vi "testScopeBasic.vi"() -> ()   [LabVIEW 2023, in "sweScope.lvlib"]
doc: "Demonstrates the usage of the Scope abstraction."
uses:
  sweScope.lvlib
  Data/scopeChnCoupling.ctl
  Data/scopeEdgeTrigger.ctl
  Data/scopeRunState.ctl
  Scope.lvclass
panel:
  out "Waveform Graph":waveform(dbl)(graph)
  out "error out":errorcluster
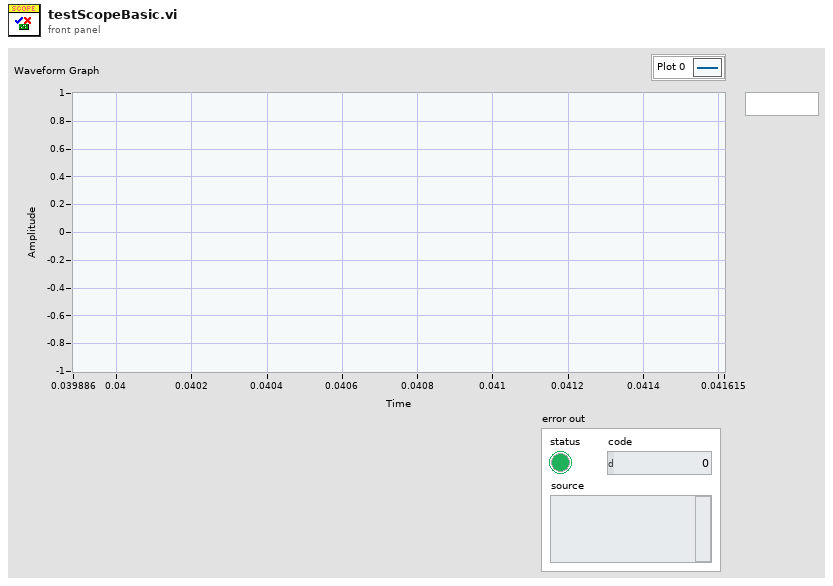
[diagram p1: front panel]
types:
  T1 = typedef "sweScope.lvlib/scopeRunState.ctl" = enum16{"AUTO", "NORMAL", "SINGLE"}
  T2 = typedef "sweScope.lvlib/scopeEdgeTrigger.ctl" = enum16{"Positive", "Negative", "Either"}
  T3 = typedef "sweScope.lvlib/scopeChnCoupling.ctl" = enum16{"DC1M", "AC1M", "DC50", "GND"}
  T4 = enum16{"Simulated", "SCOPE_NI", "SCOPE_Keysight"}
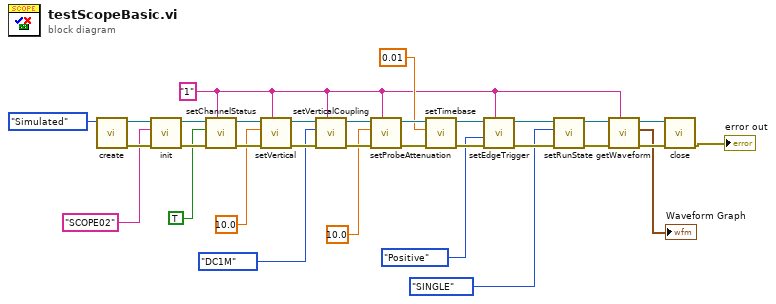
[diagram p0: block diagram]
diagram:
  w6 = "1" ("Chn")
  n1 = call "create.vi"("Type"=T4."Simulated") -> ("error out"=w31:errorcluster, "Scope.lvclass"=w32:refnum<class "Scope.lvclass">)  [unwired: 9 in]
  n2 = call-dynamic "init.vi"("error in (no error)"=w31, "Resource"="SCOPE02", "Instrument in"=w32) -> ("error out"=w29:errorcluster, "Instrument out"=w30:refnum<class "Scope.lvclass">)  [unwired: 7 in]
  n3 = call-dynamic "setChannelStatus.vi"("Chn"=w6, "error in (no error)"=w29, "State"=TRUE, "Scope in"=w30) -> ("error out"=w27:errorcluster, "Scope out"=w28:refnum<class "Scope.lvclass">)  [unwired: 6 in]
  n4 = call-dynamic "setVertical.vi"("Chn"=w6, "error in (no error)"=w27, "Range [V]"=10.0, "Scope in"=w28) -> ("error out"=w25:errorcluster, "Scope out"=w26:refnum<class "Scope.lvclass">)  [unwired: 6 in]
  n5 = call-dynamic "setVerticalCoupling.vi"("Chn"=w6, "error in (no error)"=w25, "Coupling"=scopeChnCoupling."DC1M", "Scope in"=w26) -> ("error out"=w23:errorcluster, "Scope out"=w24:refnum<class "Scope.lvclass">)  [unwired: 6 in]
  n6 = call-dynamic "setProbeAttenuation.vi"("Chn"=w6, "error in (no error)"=w23, "Attenuation"=10.0, "Scope in"=w24) -> ("error out"=w15:errorcluster, "Scope out"=w16:refnum<class "Scope.lvclass">)  [unwired: 6 in]
  n7 = call-dynamic "setTimebase.vi"("error in (no error)"=w15, "Timebase [s/Div]"=0.01, "Scope in"=w16) -> ("error out"=w13:errorcluster, "Scope out"=w14:refnum<class "Scope.lvclass">)  [unwired: 7 in]
  n8 = call-dynamic "setEdgeTrigger.vi"("Source"=w6, "error in (no error)"=w13, "Edge"=scopeEdgeTrigger."Positive", "Scope in"=w14) -> ("error out"=w11:errorcluster, "Scope out"=w12:refnum<class "Scope.lvclass">)  [unwired: 6 in]
  n9 = call-dynamic "setRunState.vi"("error in (no error)"=w11, "Runstate"=scopeRunState."SINGLE", "Scope in"=w12) -> ("error out"=w3:errorcluster, "Scope out"=w7:refnum<class "Scope.lvclass">)  [unwired: 7 in]
  n10 = call-dynamic "getWaveform.vi"("Chn"=w6, "error in (no error)"=w3, "Scope in"=w7) -> ("error out"=w4:errorcluster, "Waveform Graph"=→"Waveform Graph":waveform(dbl), "Scope out"=w5:refnum<class "Scope.lvclass">)  [unwired: 6 in]
  n11 = call-dynamic "close.vi"("error in (no error)"=w4, "Instrument in"=w5) -> ("error out"=→"error out":errorcluster)  [unwired: 9 in]
